vi "Aggregate Test Case Results.vi"(10 "Test Case Result":refnum<class "Test Case Result.lvclass">, 11 "Test Suite Result In":refnum<class "Test Suite Result.lvclass">) -> (3 "Test Suite Result Out":refnum<class "Test Suite Result.lvclass">)   [LabVIEW 2020, in "Test Suite Result.lvclass"]
uses:
  Test Suite Result.lvclass
  Test Case Result/Test Case Result.lvclass
  Test Suite Result.lvclass/Test Suite Result.ctl
  Test Case Result/Test Case Result.lvclass/Test Case Result.ctl
  Method Result/Method Result.lvclass/Method Result.ctl
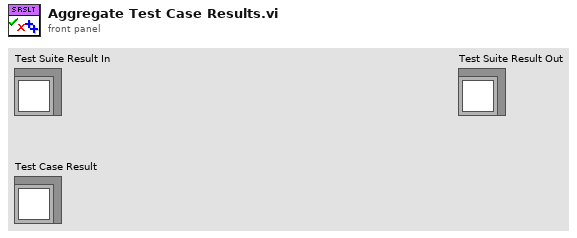
[diagram p1: front panel]
types:
  T1 = typedef "Assertion Result.lvclass/Status.ctl" = enum16{"Pass", "Fail", "Error", "Skipped", "Setup Error", "Broken", "Teardown Error"}
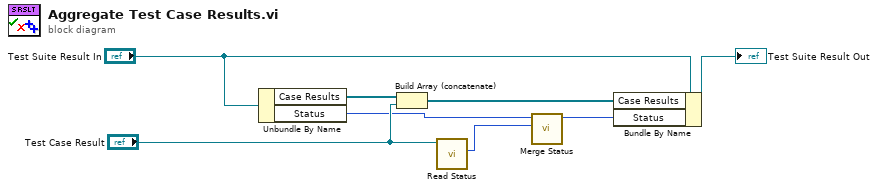
[diagram p0: block diagram]
diagram:
  n1 = Unbundle By Name("Test Suite Result In") -> ("Case Results"=w5:refnum<class "Test Case Result.lvclass">[], "Status"=w2:T1)
  n2 = Build Array (concatenate)(w5, "Test Case Result") -> (w4:refnum<class "Test Case Result.lvclass">[])
  n3 = call "Read Status.vi"("Test Case Result In"="Test Case Result") -> ("Status"=w1:T1)  [unwired: 8 in, 2 out]
  n4 = call "Merge Status.vi"("New"=w1, "Current"=w2) -> ("Merged"=w3:T1)  [unwired: 8 in, 1 out]
  n5 = Bundle By Name(cluster="Test Suite Result In", "Case Results"=w4, "Status"=w3) -> (→"Test Suite Result Out":refnum<class "Test Suite Result.lvclass">)
